vi "Find Windows.vi"(8 "error in (no error)":errorcluster, 11 "VI reference":refnum<vi>) -> (0 "error out":errorcluster, 3 "hWnd":u32)   [LabVIEW 2025, in "Test Unit.lvlib"]
uses:
  Test Unit.lvlib
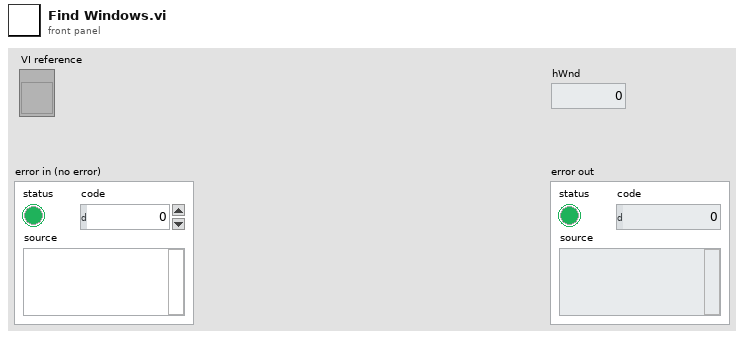
[diagram p1: front panel]
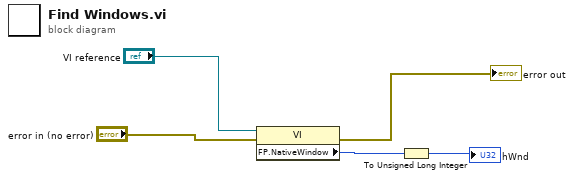
[diagram p0: block diagram]
diagram:
  n1 = property class="VI"(reference="VI reference", error in="error in (no error)") -> (error out=→"error out":errorcluster, "FP.NativeWindow"=w2:u64)  [unwired: 1 out]
  n2 = To Unsigned Long Integer(number=w2) -> (unsigned 32bit integer=→"hWnd":u32)
